vi "Teleop.vi"(10 "Match Info":T1={"Autonomous Elapsed Seconds"=0.0, "TeleOp Elapsed Seconds"=0.0, "Disabled Elapsed Seconds"=0.0, "Visited Autonomous"=FALSE, "Visited TeleOp"=FALSE, "Visited Disabled"=FALSE, "Autonomous Settings"={"Autonomous Style"=enum."Independent", "VI Refnum"=refnum}}, 11 "Call Context":T2) -> ()   [LabVIEW 2017]
doc: "This VI is called for each enabled TeleOp packet received from the DS. It is typically used to read from joysticks and other inputs and update I/O or setpoints for timed control loops. It should complete and return within 20 milliseconds or risk missing DS packets."
uses:
  <vilib>/Rock Robotics/WPI/DriverStation/WPI_DriverStationDerivedRobotMode.ctl
  <vilib>/Rock Robotics/WPI/DriverStation/WPI_DriverStationMatch Info.ctl
  <vilib>/Rock Robotics/WPI/Utilities/WPI_GetSetVariantRefNum.vi
  <vilib>/Rock Robotics/Network Tables/NT Write Boolean Array.vi
  <vilib>/Rock Robotics/Network Tables/NT Write Numeric Array.vi
panel:
  out "f 2":dbl
  out "f":dbl
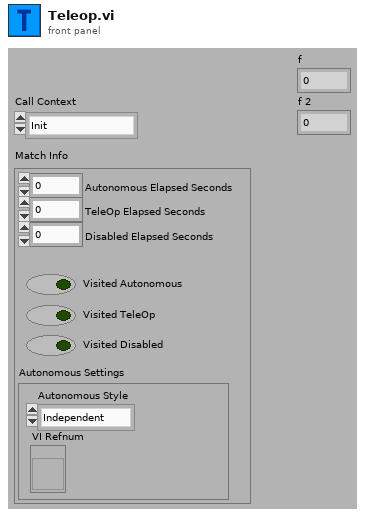
[diagram p1: front panel]
types:
  T1 = typedef "WPI_DriverStationMatch Info.ctl" = cluster{"Autonomous Elapsed Seconds":dbl, "TeleOp Elapsed Seconds":dbl, "Disabled Elapsed Seconds":dbl, "Visited Autonomous":bool, "Visited TeleOp":bool, "Visited Disabled":bool, "Autonomous Settings":cluster{"Autonomous Style":enum16{"Iterative", "Independent"}, "VI Refnum":refnum<vi>}}
  T2 = typedef "WPI_DriverStationDerivedRobotMode.ctl" = enum16{"Init", "Execute", "Stop"}
  T3 = typedef "WPI_JoystickDevRef.ctl" = cluster{"Device":T4}
  T4 = typedef "WPI_JoystickDeviceEnum.ctl" = enum16{"USB 0", "USB 1", "USB 2", "USB 3", "USB 4", "USB 5"}
  T5 = typedef "Command Status Info.ctl" = cluster{"Name":string, "Status":T6, "notifier out":T7}
  T6 = typedef "Completion Status.ctl" = enum16{"Successful", "Aborted", "Incomplete"}
  T7 = typedef "Completion Notifier.ctl" = refnum<notifier>
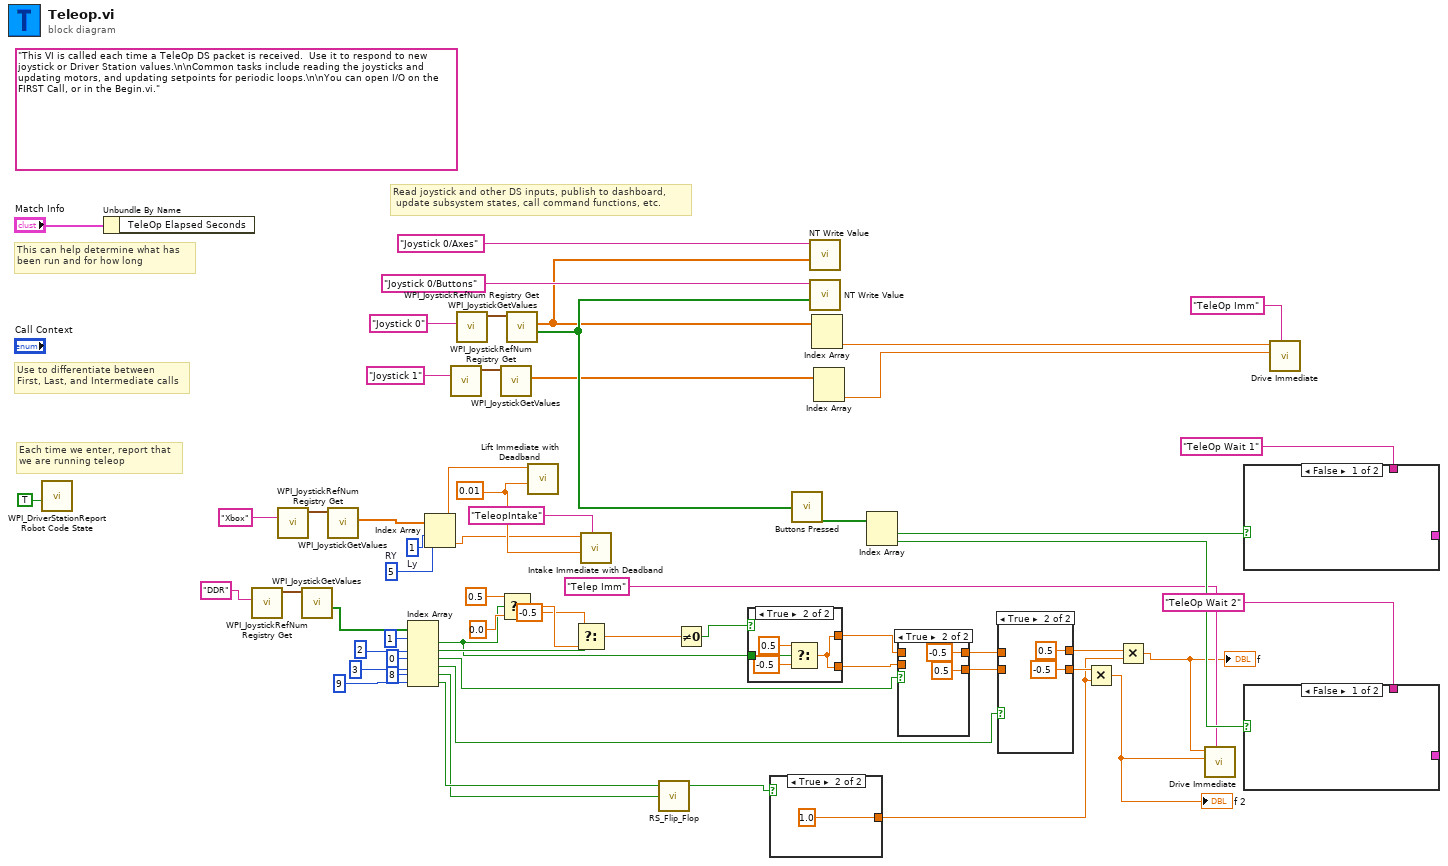
[diagram p0: block diagram]
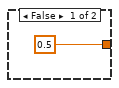
[diagram p2: hidden frame]
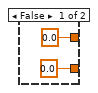
[diagram p5: hidden frame]
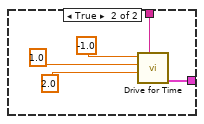
[diagram p6: hidden frame]
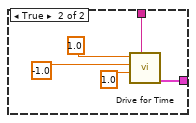
[diagram p7: hidden frame]
diagram:
  w36 = 5  # RY
  w37 = 1  # Ly
  w38 = 0.01 ("Deadband Value")
  (unwired) "This VI is called each time a TeleOp DS packet is received.  Use it to respond to new joystick or Driver Station values.\n\nCommon tasks include reading the joysticks and updating motors, and updating setpoints for periodic loops.\n\nYou can open I/O on the FIRST Call, or in the Begin.vi."
  # "Read joystick and other DS inputs, publish to dashboard,\n update subsystem states, call command functions, etc."
  # "Each time we enter, report that\nwe are running teleop"
  # "Use to differentiate between\nFirst, Last, and Intermediate calls"
  # "This can help determine what has\nbeen run and for how long"
  n1 = call <vilib>:"WPI_DriverStationReport Robot Code State.vi"("TeleOp"=TRUE ("Autonomous")) -> ()  [unwired: 10 in, 1 out]
  n2 = Unbundle By Name("Match Info") -> ()  [unwired: 1 out]
  n3 = call <vilib>:"WPI_JoystickRefNum Registry Get.vi"("refnum name"="DDR") -> ("JoystickDevRef"=w31:T3)  [unwired: 1 in, 9 out]
  n4 = call <vilib>:"WPI_JoystickRefNum Registry Get.vi"("refnum name"="Xbox") -> ("JoystickDevRef"=w41:T3)  [unwired: 1 in, 9 out]
  n5 = call <vilib>:"WPI_JoystickGetValues.vi"("JoystickDevRef"=w31) -> ("Buttons"=w30:bool[])  [unwired: 6 in, 4 out]
  n6 = call <vilib>:"WPI_JoystickGetValues.vi"("JoystickDevRef"=w41) -> ("Axes"=w40:dbl[])  [unwired: 6 in, 4 out]
  n7 = Index Array(array=w30, index #1=2 ("index"), index #2=1 ("index"), index #3=0 ("index"), index #4=3 ("index"), index #5=8 ("index"), index #6=9 ("index")) -> (element #1=w11:bool, element #2=w25:bool, element #3=w15:bool, element #4=w12:bool, element #5=w7:bool, element #6=w8:bool)
  n8 = Index Array(array=w40, index #1=w37, index #2=w36) -> (element #1=w35:dbl, element #2=w34:dbl)
  n9 = call <vilib>:"WPI_JoystickRefNum Registry Get.vi"("refnum name"="Joystick 1") -> ("JoystickDevRef"=w46:T3)  [unwired: 1 in, 9 out]
  n10 = call <vilib>:"WPI_JoystickRefNum Registry Get.vi"("refnum name"="Joystick 0") -> ("JoystickDevRef"=w57:T3)  [unwired: 1 in, 9 out]
  n11 = call <vilib>:"WPI_JoystickGetValues.vi"("JoystickDevRef"=w46) -> ("Axes"=w45:dbl[])  [unwired: 6 in, 4 out]
  n12 = Select(t=0.5, s=w11, f=0.0) -> (s? t:f=w22:dbl)
  n13 = call <vilib>:"WPI_JoystickGetValues.vi"("JoystickDevRef"=w57) -> ("Buttons"=w50:bool[], "Axes"=w49:dbl[])  [unwired: 6 in, 3 out]
  n14 = call "Lift Immediate with Deadband.vi"("Deadband Value"=w38, "Setpoint"=w35) -> ()  [unwired: 9 in, 1 out]
  n15 = Select(t=-0.5, s=w25, f=w22) -> (s? t:f=w18:dbl)
  n16 = call "Intake Immediate with Deadband.vi"("Description"="TeleopIntake", "Deadband Value"=w38, "Setpoint"=w34) -> ()  [unwired: 8 in, 1 out]
  n17 = call "RS_Flip_Flop.vi"("Set"=w7, "Reset"=w8) -> ("Q"=w6:bool)  [unwired: 1 in, 2 out]
  n18 = Not Equal To 0?(x=w18) -> (x != 0?=w19:bool)
  n19 = case shown="True" w19 {
    tunnel: [0.0 w64] -> w16
    tunnel: [0.0 w64] -> w17
    tunnel: w11 -> [_ w63]
    frame False {
    }
    frame True {
      n20 = Select(t=0.5, s=w63, f=-0.5) -> (s? t:f=w64:dbl)
    }
  }
  n21 = case shown="True" w6 {
    tunnel: [0.5 1.0] -> w1
    frame False {
    }
    frame True {
    }
  }
  n22 = call "Buttons Pressed.vi"("Button Values"=w50) -> ("Button Presses"=w54:bool[])
  n23 = call-poly <vilib>:"NT Write Value.vi"("Numeric Array"=w49, "Name"="Joystick 0/Axes") -> ()  [unwired: 9 in, 1 out]
  n24 = call-poly <vilib>:"NT Write Value.vi"("Boolean Array"=w50, "Name"="Joystick 0/Buttons") -> ()  [unwired: 9 in, 1 out]
  n25 = Index Array(array=w49) -> (element #2=w43:dbl)  [unwired: 2 in, 1 out]
  n26 = Index Array(array=w45) -> (element #2=w44:dbl)  [unwired: 2 in, 1 out]
  n27 = Index Array(array=w54) -> (element #1=w53:bool, element #2=w52:bool)  [unwired: 2 in]
  n28 = case shown="True" w15 {
    tunnel: w17 -> [w70 _]
    tunnel: w16 -> [w69 _]
    tunnel: [w70 -0.5 ("f")] -> w14
    tunnel: [w69 0.5 ("f")] -> w13
    frame False {
    }
    frame True {
    }
  }
  n29 = case shown="True" w12 {
    tunnel: w14 -> [w74 _]
    tunnel: w13 -> [w73 _]
    tunnel: [w74 0.5 ("f")] -> w5
    tunnel: [w73 -0.5 ("f")] -> w4
    frame False {
    }
    frame True {
    }
  }
  n30 = Multiply(x=w4, y=w1) -> (x*y=w2:dbl)
  "f 2" <- w2
  n31 = Multiply(x=w5, y=w1) -> (x*y=w3:dbl)
  "f" <- w3
  n32 = call "Drive Immediate.vi"("Description"="Telep Imm", "Right Setpoint"=w2, "Left Setpoint"=w3) -> ()  [unwired: 8 in, 1 out]
  n33 = case shown="False" w53 {
    tunnel: [_ w80] -> _
    tunnel: "TeleOp Wait 1" ("Description") -> [_ w79]
    frame False {
    }
    frame True {
      n34 = call "Drive for Time.vi"("Description"=w79, "Seconds"=1.0, "Right Speed"=-1.0, "Left Speed"=1.0) -> ("Command Info Out"=w80:T5)  [unwired: 6 in, 1 out]
    }
  }
  n35 = case shown="False" w52 {
    tunnel: [_ w84] -> _
    tunnel: "TeleOp Wait 2" ("Description") -> [_ w83]
    frame False {
    }
    frame True {
      n36 = call "Drive for Time.vi"("Description"=w83, "Seconds"=2.0, "Right Speed"=1.0, "Left Speed"=-1.0) -> ("Command Info Out"=w84:T5)  [unwired: 6 in, 1 out]
    }
  }
  n37 = call "Drive Immediate.vi"("Description"="TeleOp Imm", "Right Setpoint"=w44, "Left Setpoint"=w43) -> ()  [unwired: 8 in, 1 out]
